vi "SP Update Markers in Plots.vi"(5 "CH Control":T1={"Trace Orientation"=enum."Overlay", "Frequency"={"Change Frequency"=FALSE, "Start"=500.0, "Stop"=1500.0, "Units"=enum."MHz"}, "Markers"=[], "Traces"=[]} {"Traces"."Reference" format="%#.2g"; "Traces"."Display Data" items=["Data", "Memory", "Data/Memory"]; "Traces"."Format" items=["Log Mag", "Phase", "Expanded Phase", "Delay", "Smith", "Polar", "Lin Mag", "SWR", "Loss", "Real", "Imaginary"]; "Traces"."Scale" min=0.001 step=1.0 format="%#.2g"; "Traces"."Position" min=0.0 max=10.0; "Frequency"."Stop" format="%.3g"; "Frequency"."Start" format="%.3g"}, 7 "Plot References":refnum<vi>[](array[refnum]), 8 "error in (no error)":errorcluster, 11 "Plot Ref":refnum<vi>) -> (0 "error out":errorcluster)   [LabVIEW 2011]
uses:
  TypeDefs/SP Display Plot Controls Cluster.ctl
  TypeDefs/SP Frequency Units.ctl
  TypeDefs/SP Marker Cluster.ctl
  TypeDefs/SP Marker Type.ctl
  TypeDefs/SP Display Trace Controls.ctl
  TypeDefs/SP Display Format.ctl
  TypeDefs/SP Display Data.ctl
panel:
  # "Div"
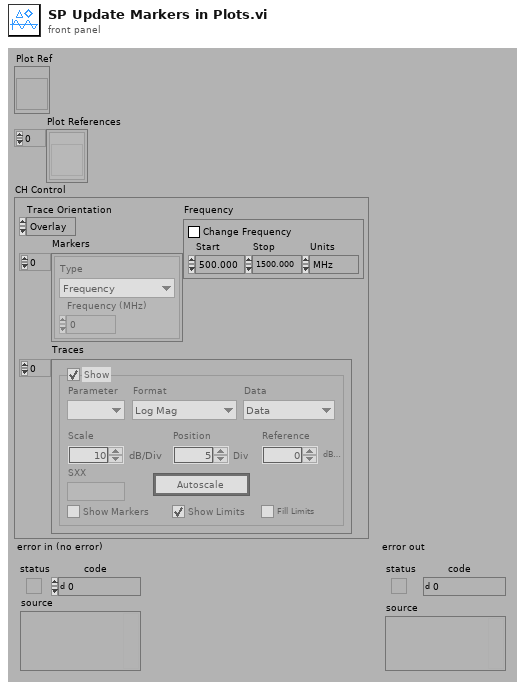
[diagram p1: front panel]
types:
  T1 = typedef "SP Display Plot Controls Cluster.ctl" = cluster{"Trace Orientation":enum32{"Overlay", "Split"}, "Frequency":cluster{"Change Frequency":bool, "Start":dbl, "Stop":dbl, "Units":T2}, "Markers":T3[], "Traces":T5[]}
  T2 = typedef "SP Frequency Units.ctl" = enum16{"Hz", "kHz", "MHz", "GHz", "Points"}
  T3 = typedef "SP Marker Cluster.ctl" = cluster{"Type":T4, "Frequency (MHz)":dbl}
  T4 = typedef "SP Marker Type.ctl" = enum16{"Frequency", "Trace Maximum", "Trace Minimum", "Limit Maximum", "Limit Minimum"}
  T5 = typedef "SP Display Trace Controls.ctl" = cluster{"Trace On":bool, "Measure":i32, "Format":T6, "Autoscale":bool, "Reference":dbl, "\nRefUnit":string, "Position":dbl, "Scale":dbl, "ScaleUnit":string, "LimitOn":bool, "LimitFill":bool, "Display Data":T7, "Show Markers":bool, "SXX":string}
  T6 = typedef "SP Display Format.ctl" = i32
  T7 = typedef "SP Display Data.ctl" = u16
  T8 = typedef "SP Channel Data.ctl" = cluster{"Graph Ref":refnum<vi>, "Data":cluster{"Data":cluster{"X":dbl[], "Y":dbl[]}, "Index":i32}, "ULimits":cluster{"Data":cluster{"X":dbl[], "Y":dbl[]}, "Index":i32}[], "LLimits":cluster{"Data":cluster{"X":dbl[], "Y":dbl[]}, "Index":i32}[]}
  T9 = typedef "LVCursorListTypeDef.ctl" = cluster{"Name":string, "Color":u32, "Style":u8, "Point Style":u8, "Name Visible":bool, "Allow Drag":bool, "Cursor Mode":u32, "Plot":i32, "Index":i32, "Position":cluster{"X":dbl, "Y":dbl}, "X Scale":u32, "Y Scale":u32, "Watch Plots":i32[], "Watch All Plots":bool, "Plot Area":i32, "Label Offset":cluster{"X":dbl, "Y":dbl}}[]
  T10 = cluster{"Name":string, "Color":u32, "Style":u8, "Point Style":u8, "Name Visible":bool, "Allow Drag":bool, "Cursor Mode":u32, "Plot":i32, "Index":i32, "Position":cluster{"X":dbl, "Y":dbl}, "X Scale":u32, "Y Scale":u32, "Watch Plots":i32[], "Watch All Plots":bool, "Plot Area":i32, "Label Offset":cluster{"X":dbl, "Y":dbl}}
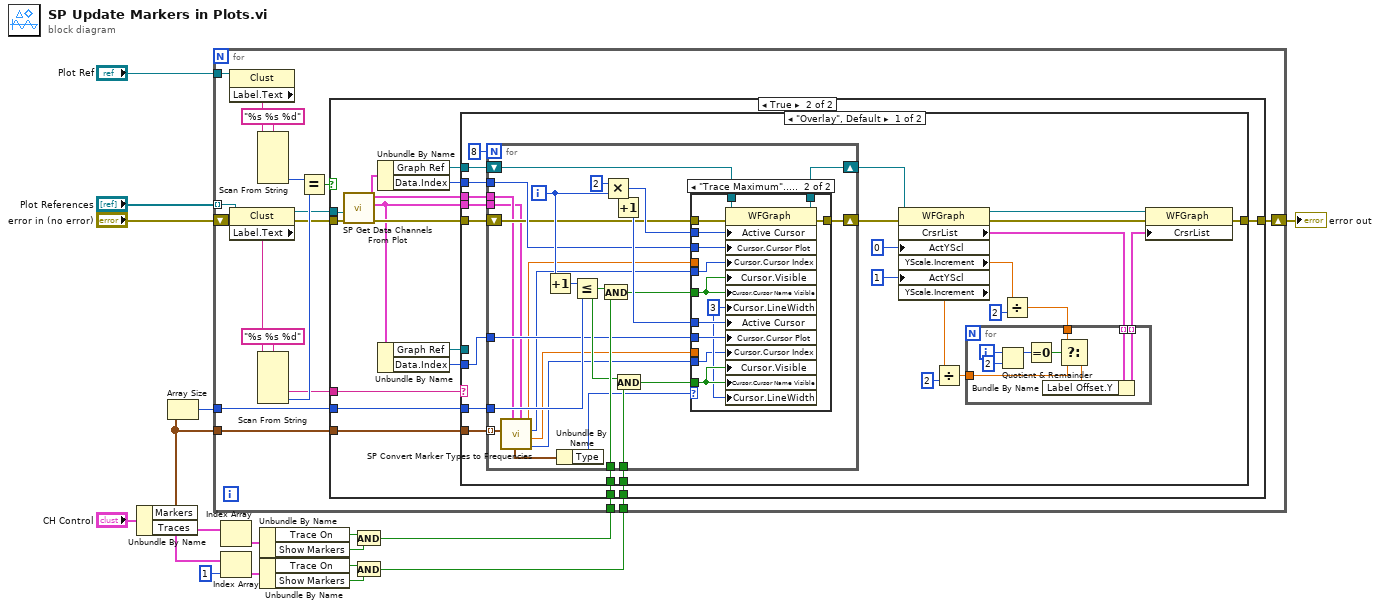
[diagram p0: block diagram]
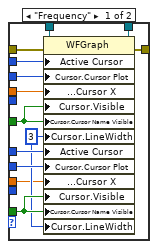
[diagram p3: hidden frame]
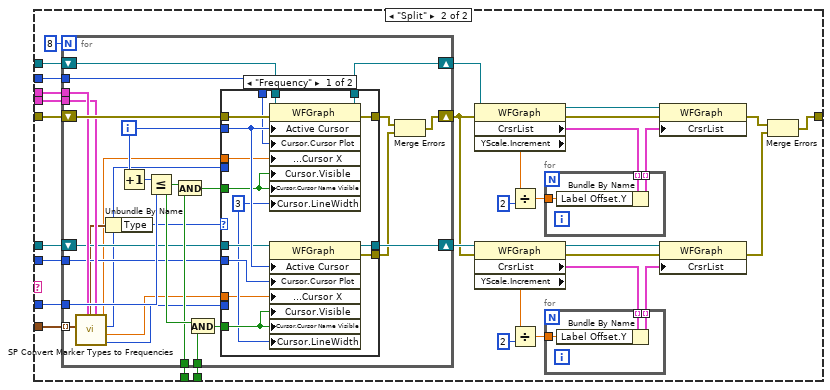
[diagram p4: hidden frame]
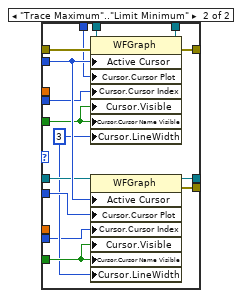
[diagram p5: hidden frame]
diagram:
  n1 = Unbundle By Name("CH Control") -> ("Markers"=w2:T3[], "Traces"=w7:T5[])
  n2 = Array Size(array=w2) -> (size(s)=w13:i32)
  n3 = Index Array(array=w7) -> (element=w10:T5)  [unwired: 1 in]
  n4 = Index Array(array=w7, index=1) -> (element=w9:T5)
  n5 = Unbundle By Name(w10) -> ("Trace On"=w6:bool, "Show Markers"=w3:bool)
  n6 = Unbundle By Name(w9) -> ("Trace On"=w5:bool, "Show Markers"=w4:bool)
  n7 = And(x=w6, y=w3) -> (x .and. y?=w12:bool)
  n8 = And(x=w5, y=w4) -> (x .and. y?=w11:bool)
  n9 = for {
    tunnel: w2 -> [w34]
    tunnel: "Plot Ref" -> [w27]
    tunnel: "Plot References" -> [w24] mode=indexing
    shift-right: [w35] -> w17
    shift-left: "error in (no error)" -> [w26]
    tunnel: w13 -> [w20]
    tunnel: w12 -> [w19]
    tunnel: w11 -> [w18]
    n10 = property class="Clust"(reference=w27) -> ("Label.Text"=w30:string)  [unwired: 1 in, 2 out]
    n11 = property class="Clust"(reference=w24, error in=w26) -> (reference out=w23:refnum<vi>, error out=w25:errorcluster, "Label.Text"=w32:string)
    n12 = Scan From String(format string="%s %s %d", input string=w30) -> (output 3=w29:i32)  [unwired: 2 in, 8 out]
    n13 = Scan From String(format string="%s %s %d", input string=w32) -> (output 2=w21:string, output 3=w28:i32)  [unwired: 2 in, 7 out]
    n14 = Equal?(x=w29, y=w28) -> (x = y?=w22:bool)
    n15 = case shown="True" w22 {
      tunnel: [w36 w51] -> w35
      tunnel: w34 -> [_ w50]
      tunnel: w25 -> [w36 w47]
      tunnel: w23 -> [_ w48]
      tunnel: w21 -> [_ w49]
      tunnel: w20 -> [_ w45]
      tunnel: w19 -> [_ w44]
      tunnel: w18 -> [_ w43]
      frame False {
      }
      frame True {
        n16 = call "SP Get Data Channels From Plot.vi"("error in (no error)"=w47, "Plot Ref"=w48) -> ("error out"=w46:errorcluster, "CH 2"=w39:T8, "CH 1"=w42:T8)  [unwired: 7 out]
        n17 = Unbundle By Name(w42) -> ("Graph Ref"=w41:refnum<vi>, "Data.Index"=w40:i32)
        n18 = Unbundle By Name(w39) -> ("Graph Ref"=w37:refnum<vi>, "Data.Index"=w38:i32)
        n19 = case shown="\"Overlay\", Default" w49 {
          tunnel: [w64 w141] -> w51
          tunnel: w50 -> [w70 w162]
          tunnel: w46 -> [w75 w167]
          tunnel: w39 -> [w76 w168]
          tunnel: w42 -> [w77 w169]
          tunnel: w45 -> [w74 w165]
          tunnel: w44 -> [w72 w163]
          tunnel: w43 -> [w71 w164]
          tunnel: w41 -> [w53 w161]
          tunnel: w40 -> [w69 w160]
          tunnel: w38 -> [w68 w158]
          tunnel: w37 -> [_ w159]
          frame "Overlay", Default {
            n20 = for {
              N: 8 -> [_]
              tunnel: w77 -> [w95]
              tunnel: w76 -> [w94]
              shift-right: [w96] -> w63
              shift-left: w75 -> [w98]
              tunnel: w74 -> [w108]
              tunnel: w72 -> [w107]
              tunnel: w71 -> [w105]
              tunnel: w70 -> [w93] mode=indexing
              tunnel: w69 -> [w100]
              tunnel: w68 -> [w99]
              shift-right: [w87] -> w52
              shift-left: w53 -> [w97]
              i -> [w102]
              n21 = call "SP Convert Marker Types to Frequencies.vi"("CH 2"=w94, "CH 1"=w95, "Marker"=w93) -> ("CH2 Index"=w88:i32, "CH2 Frequency"=w89:dbl, "CH1 Index"=w90:i32, "CH1 Frequency"=w91:dbl)  [unwired: 3 out]
              n22 = Increment(x=w102) -> (x+1=w109:i32)
              n23 = Unbundle By Name(w93) -> ("Type"=w92:T4)
              n24 = Less Or Equal?(x=w109, y=w108) -> (x <= y?=w104:bool)
              n25 = And(x=w104, y=w107) -> (x .and. y?=w106:bool)
              n26 = Multiply(x=2 ("y"), y=w102) -> (x*y=w110:i32)
              n27 = Increment(x=w110) -> (x+1=w111:i32)
              n28 = And(x=w104, y=w105) -> (x .and. y?=w101:bool)
              n29 = case shown="\"Trace Maximum\"..\"Limit Minimum\"" w92 {
                tunnel: w111 -> [w124 w137]
                tunnel: w110 -> [w123 w136]
                tunnel: w106 -> [w122 w135]
                tunnel: w101 -> [w121 w134]
                tunnel: w100 -> [w120 w133]
                tunnel: w99 -> [w119 w132]
                tunnel: w98 -> [w118 w131]
                tunnel: w97 -> [w117 w130]
                tunnel: [w116 w129] -> w96
                tunnel: w91 -> [w114 _]
                tunnel: w89 -> [w113 _]
                tunnel: w90 -> [_ w127]
                tunnel: w88 -> [_ w126]
                tunnel: [w112 w125] -> w87
                frame "Frequency" {
                  w115 = u8 3 ("Cursor.Line Width")
                  n30 = property class="WFGraph"(reference=w117, error in=w118, "Active Cursor"=w123, "Cursor.Cursor Plot"=w120, "Cursor.Cursor Position:Cursor X"=w114, "Cursor.Visible"=w122, "Cursor.Cursor Name Visible"=w122, "Cursor.LineWidth"=w115, "Active Cursor"=w124, "Cursor.Cursor Plot"=w119, "Cursor.Cursor Position:Cursor X"=w113, "Cursor.Visible"=w121, "Cursor.Cursor Name Visible"=w121, "Cursor.LineWidth"=w115) -> (reference out=w112:refnum<vi>, error out=w116:errorcluster)
                }
                frame "Trace Maximum".."Limit Minimum" {
                  w128 = u8 3 ("Cursor.Line Width")
                  n31 = property class="WFGraph"(reference=w130, error in=w131, "Active Cursor"=w136, "Cursor.Cursor Plot"=w133, "Cursor.Cursor Index"=w127, "Cursor.Visible"=w135, "Cursor.Cursor Name Visible"=w135, "Cursor.LineWidth"=w128, "Active Cursor"=w137, "Cursor.Cursor Plot"=w132, "Cursor.Cursor Index"=w126, "Cursor.Visible"=w134, "Cursor.Cursor Name Visible"=w134, "Cursor.LineWidth"=w128) -> (reference out=w125:refnum<vi>, error out=w129:errorcluster)
                }
              }
            }
            n32 = property class="WFGraph"(reference=w52, error in=w63, "ActYScl"=0 ("Active Y Scale"), "ActYScl"=1 ("Active Y Scale")) -> (reference out=w66:refnum<vi>, error out=w65:errorcluster, "CrsrList"=w62:T9, "YScale.Increment"=w58:dbl, "YScale.Increment"=w56:dbl)
            n33 = Divide(x=w56, y=2) -> (x/y=w54:dbl)
            n34 = Divide(x=w58, y=2) -> (x/y=w55:dbl)
            n35 = for {
              tunnel: w62 -> [w86] mode=indexing
              tunnel: [w85] -> w61 mode=indexing
              tunnel: w55 -> [w79]
              tunnel: w54 -> [w78]
              i -> [w84]
              n36 = Quotient & Remainder(x=w84, y=2) -> (x-y*floor(x/y)=w82:i32)  [unwired: 1 out]
              n37 = Equal To 0?(x=w82) -> (x = 0?=w81:bool)
              n38 = Select(t=w79, s=w81, f=w78) -> (s? t:f=w80:dbl)
              n39 = Bundle By Name(cluster=w86, "Label Offset.Y"=w80) -> (w85:T10)
            }
            n40 = property class="WFGraph"(reference=w66, error in=w65, "CrsrList"=w61) -> (error out=w64:errorcluster)  [unwired: 1 out]
          }
          frame "Split" {
            n41 = for {
              N: 8 -> [_]
              tunnel: w169 -> [w192]
              tunnel: w168 -> [w191]
              shift-right: [w185] -> w155
              shift-left: w167 -> [w201]
              tunnel: w165 -> [w196]
              tunnel: w164 -> [w198]
              tunnel: w163 -> [w197]
              tunnel: w162 -> [w182] mode=indexing
              tunnel: w160 -> [w189]
              tunnel: w158 -> [w187]
              shift-right: [w186] -> w157
              shift-left: w159 -> [w188]
              shift-right: [w176] -> w156
              shift-left: w161 -> [w190]
              i -> [w195]
              n42 = call "SP Convert Marker Types to Frequencies.vi"("CH 2"=w191, "CH 1"=w192, "Marker"=w182) -> ("CH2 Index"=w178:i32, "CH2 Frequency"=w179:dbl, "CH1 Index"=w177:i32, "CH1 Frequency"=w180:dbl)  [unwired: 3 out]
              n43 = Unbundle By Name(w182) -> ("Type"=w181:T4)
              n44 = Increment(x=w195) -> (x+1=w200:i32)
              n45 = Less Or Equal?(x=w200, y=w196) -> (x <= y?=w199:bool)
              n46 = And(x=w199, y=w197) -> (x .and. y?=w194:bool)
              n47 = And(x=w199, y=w198) -> (x .and. y?=w193:bool)
              n48 = case shown="\"Frequency\"" w181 {
                tunnel: w201 -> [w216 w231]
                tunnel: w195 -> [w215 w230]
                tunnel: w194 -> [w214 w229]
                tunnel: w193 -> [w213 w228]
                tunnel: w190 -> [w212 w227]
                tunnel: w189 -> [w211 w226]
                tunnel: w188 -> [w210 w225]
                tunnel: w187 -> [w209 w224]
                tunnel: [w207 w222] -> w186
                tunnel: [w206 w221] -> w184
                tunnel: [w205 w220] -> w183
                tunnel: w180 -> [w204 _]
                tunnel: w179 -> [w203 _]
                tunnel: w178 -> [_ w219]
                tunnel: w177 -> [_ w218]
                tunnel: [w202 w217] -> w176
                frame "Frequency" {
                  w208 = u8 3 ("Cursor.Line Width")
                  n49 = property class="WFGraph"(reference=w212, error in=w216, "Active Cursor"=w215, "Cursor.Cursor Plot"=w211, "Cursor.Cursor Position:Cursor X"=w204, "Cursor.Visible"=w214, "Cursor.Cursor Name Visible"=w214, "Cursor.LineWidth"=w208) -> (reference out=w202:refnum<vi>, error out=w206:errorcluster)
                  n50 = property class="WFGraph"(reference=w210, "Active Cursor"=w215, "Cursor.Cursor Plot"=w209, "Cursor.Cursor Position:Cursor X"=w203, "Cursor.Visible"=w213, "Cursor.Cursor Name Visible"=w213, "Cursor.LineWidth"=w208) -> (reference out=w207:refnum<vi>, error out=w205:errorcluster)  [unwired: 1 in]
                }
                frame "Trace Maximum".."Limit Minimum" {
                  w223 = u8 3 ("Cursor.Line Width")
                  n51 = property class="WFGraph"(reference=w227, error in=w231, "Active Cursor"=w230, "Cursor.Cursor Plot"=w226, "Cursor.Cursor Index"=w218, "Cursor.Visible"=w229, "Cursor.Cursor Name Visible"=w229, "Cursor.LineWidth"=w223) -> (reference out=w217:refnum<vi>, error out=w221:errorcluster)
                  n52 = property class="WFGraph"(reference=w225, "Active Cursor"=w230, "Cursor.Cursor Plot"=w224, "Cursor.Cursor Index"=w219, "Cursor.Visible"=w228, "Cursor.Cursor Name Visible"=w228, "Cursor.LineWidth"=w223) -> (reference out=w222:refnum<vi>, error out=w220:errorcluster)  [unwired: 1 in]
                }
              }
              n53 = Merge Errors(w184, w183) -> (w185:errorcluster)
            }
            n54 = property class="WFGraph"(reference=w156, error in=w155) -> (reference out=w149:refnum<vi>, error out=w150:errorcluster, "CrsrList"=w152:T9, "YScale.Increment"=w138:dbl)
            n55 = property class="WFGraph"(reference=w157, error in=w155) -> (reference out=w148:refnum<vi>, error out=w147:errorcluster, "CrsrList"=w143:T9, "YScale.Increment"=w144:dbl)
            n56 = Divide(x=w138, y=2) -> (x/y=w153:dbl)
            n57 = Divide(x=w144, y=2) -> (x/y=w146:dbl)
            n58 = for {
              tunnel: w152 -> [w175] mode=indexing
              tunnel: w153 -> [w174]
              tunnel: [w173] -> w151 mode=indexing
              n59 = Bundle By Name(cluster=w175, "Label Offset.Y"=w174) -> (w173:T10)
            }
            n60 = for {
              tunnel: w143 -> [w172] mode=indexing
              tunnel: w146 -> [w171]
              tunnel: [w170] -> w142 mode=indexing
              n61 = Bundle By Name(cluster=w172, "Label Offset.Y"=w171) -> (w170:T10)
            }
            n62 = property class="WFGraph"(reference=w149, error in=w150, "CrsrList"=w151) -> (error out=w140:errorcluster)  [unwired: 1 out]
            n63 = property class="WFGraph"(reference=w148, error in=w147, "CrsrList"=w142) -> (error out=w139:errorcluster)  [unwired: 1 out]
            n64 = Merge Errors(w140, w139) -> (w141:errorcluster)
          }
        }
      }
    }
  }
  "error out" <- w17
